vi "MIMIC Commands Rev 3.vi"(6 "MIMIC HOST COMMAND":T2(ring)=enum."Read Serial Number", 8 "Input String Data Array":string[](array[string])=["1"], 9 "HWHSflag":bool, 10 "wait (ms)":u32=500, 11 "VISA resource name":refnum<visa-resource-name>="COM5") -> (0 "error out":errorcluster={"status"=FALSE, "code"=1073676294, "source"="VISA Read in MIMIC RecvCommand.vi->MIMIC Commands Rev 2.vi"}, 1 "Receive_buffer":u8[](array[numeric]) format="%x", 2 "Receive_Unpacked_Data":T1)   [LabVIEW 2014]
panel:
  out "Array 2":u8[](array[numeric])
  out "Array":u8[](array[numeric])
  out "TimeToDecode":u16
  out "VISA resource name OUT":refnum<visa-resource-name>="COM5"
  out "hex integer string":string[](array[string])=["4", "D0", "0", "0", "FF", "2C"]
types:
  T1 = cluster{"Code_Revision":string, "Decode_Data":string, "Decode_Status":string, "Response_String_1":string, "Response_String_2":string, "Response_String_3":string, "Response_String_4":string, "Response_String_5":string, "Response_String_6":string, "Time_To_Decode":u16}
  T2 = enum16{"Enter FAT", "Beeper Control", "LED Off", "LED On", "Image Mode", "Start Session", "Stop Session", "Change Buadrate", "Auto Exposure", "Set Manual Exposure", "Read BT Address", "Store BT Address", "Pairing Command", "Query Paired Address", "Pairing Status", "Un-Pairing", "Set Illumination", "Trigger", "Set Defaults", "Imager Time To Decode Test", "Battery Off", "Battery Charge Control", "Read Battery Voltage", "Read Battery Temperature", "Software Version", "StoreFeatureSet", "ReadFeatureSet", "Store Model Number", "Read Model Number", "Store Manufacturing Date", "Read Manufacturing Date", "Store Service Date", "Read Service Date", "Store Serial Number", "Read Serial Number", "Exit FAT", "Read GUID", "Cable Auto ID", "Store RSM 627", "Read RSM 627", "Hall Effect switch", "ReadObjectSensor_AD", "Store_IR_Calibration", "Read_IR_Calibration", "Aim On", "Aim Off"}
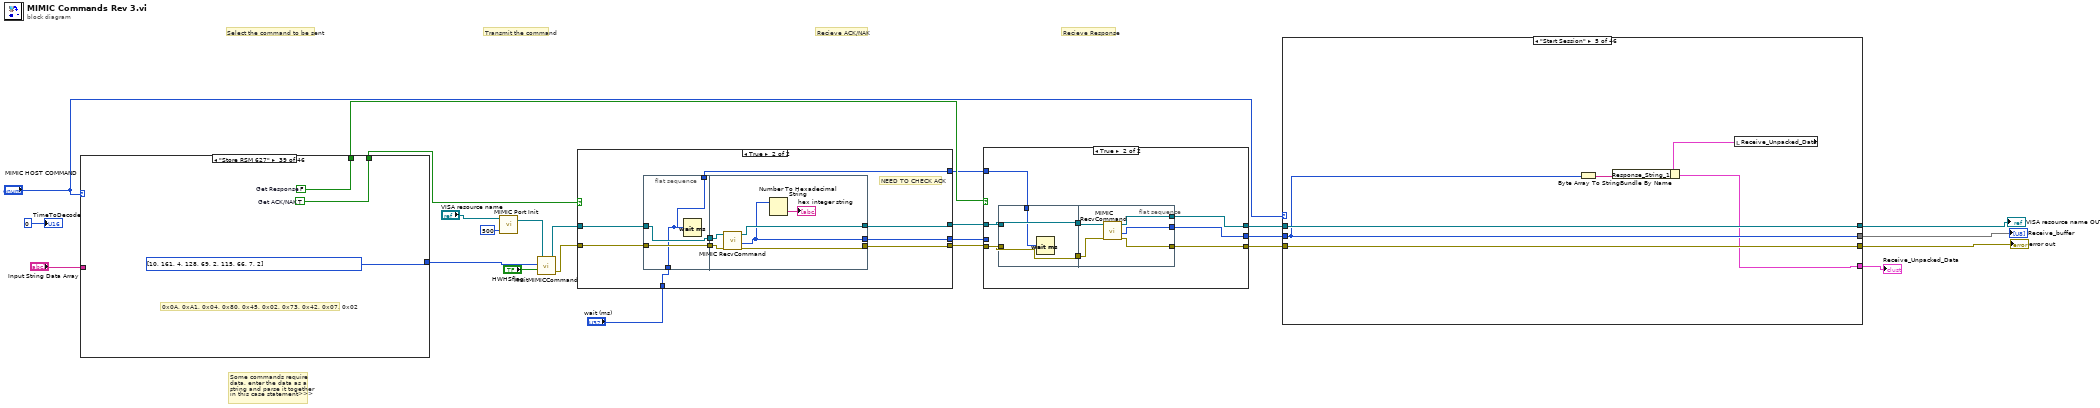
[diagram p0: block diagram]
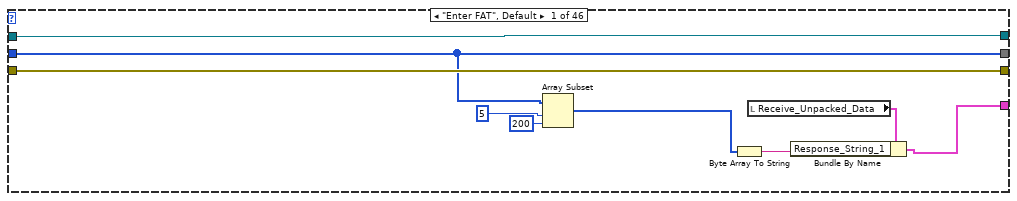
[diagram p2: hidden frame]
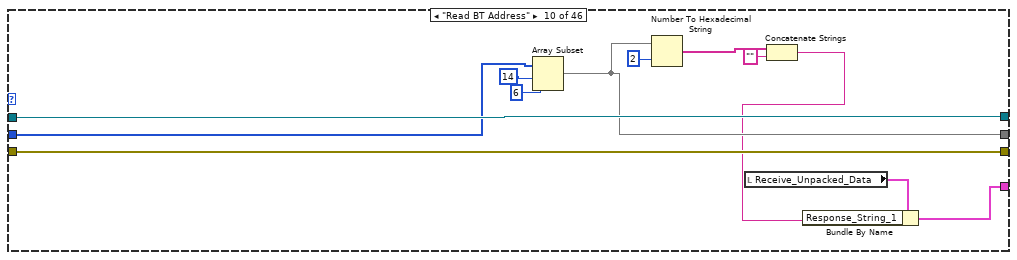
[diagram p10: hidden frame]
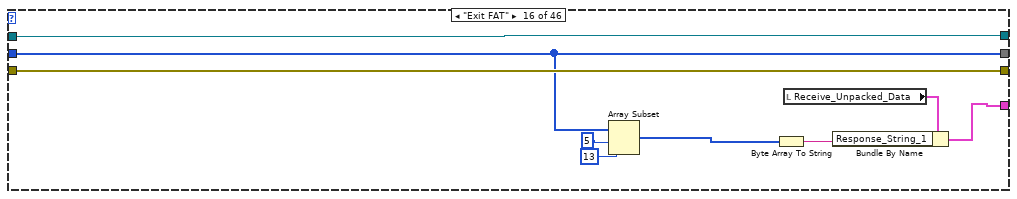
[diagram p16: hidden frame]
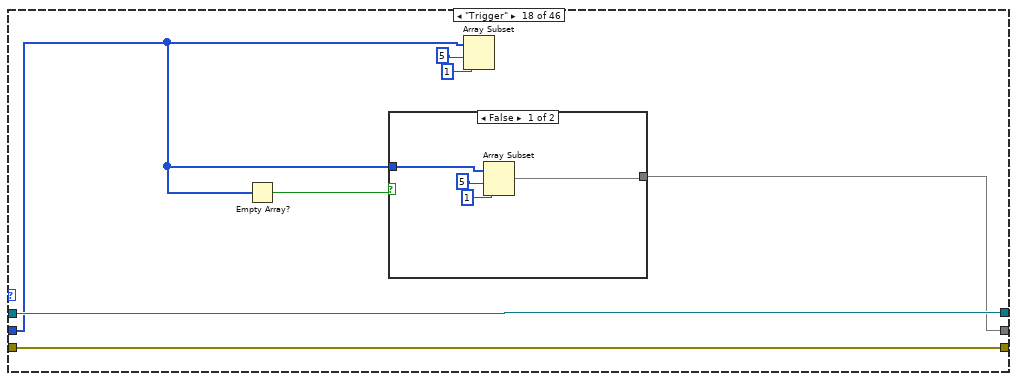
[diagram p18: hidden frame]
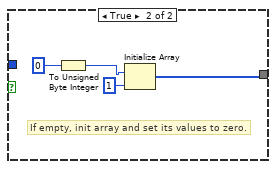
[diagram p19: hidden frame]
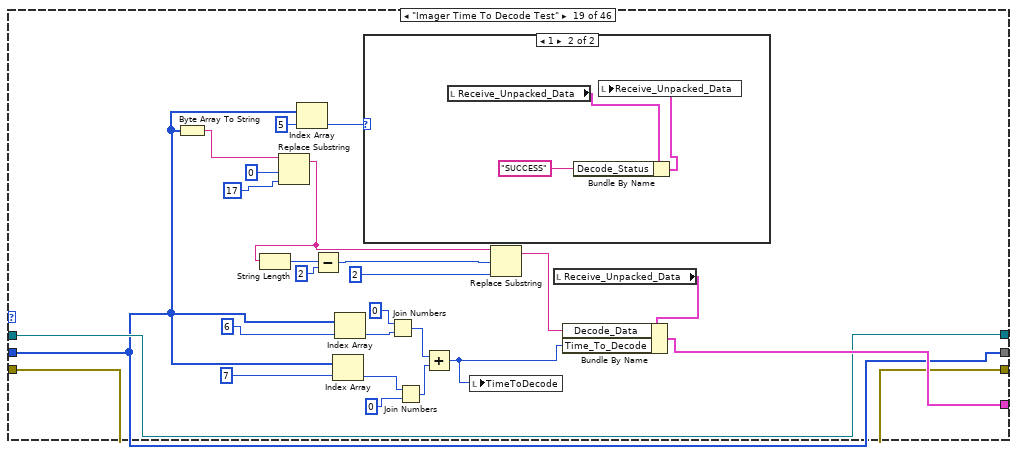
[diagram p20: hidden frame]
diagram:
  # "Transmit the command"
  # "Recieve Response"
  # "Recieve ACK/NAK"
  # "Select the command to be sent"
  # "Some commands require\ndata, enter the data as a\nstring and parse it together\nin this case statement>>>"
  n1 = case shown="\"Store RSM 627\"" "MIMIC HOST COMMAND" {
    tunnel: "Input String Data Array" -> [w33 w34 _ w45 _ _ _ w63 w79 w89 w102 _ _ _ _ _ w126 _ _ _ w146 _ _ _ w163 _ w173 _ _ _ w199 _ w211 _ _ _ _ _ _ _ _ _ w246 _ _ _]
    tunnel: [w27 w38 u8[] [5, 161, 4, 128, 16, 0, 0, 0, 0, 0, 0, 0, 0, 0] w46 u8[] [4, 228, 4, 0, 0, 0, 0, 0, 0, 0, 0, 0, 0, 0] u8[] [4, 228, 4, 0, 0, 0, 0, 0, 0, 0, 0, 0, 0, 0] u8[] [7, 215, 4, 0, 4, 11, 0, 255, 15, 0, 0, 0, 0, 0] w64 w73 w87 w101 u8[] [16, 161, 4, 128, 16, 0, 0, 0, 0, 0, 0, 0, 0, 0] u8[] [5, 161, 4, 128, 16, 0, 0, 0, 0, 0, 0, 0, 0, 0] u8[] [4, 200, 4, 128, 0, 0, 0, 0, 0, 0, 0, 0, 0, 0] u8[] [5, 161, 4, 128, 25, 0, 0, 0, 0, 0, 0, 0, 0, 0] u8[] [7, 161, 4, 128, 66, 2, 29, 0, 0, 0, 0, 0, 0, 0] w125 u8[] [6, 161, 4, 128, 45, 2, 0, 0, 0, 0, 0, 0, 0, 0] u8[] [7, 161, 4, 128, 48, 19, 136, 0, 0, 0, 0, 0, 0, 0] u8[] [5, 161, 4, 128, 60, 0, 0, 0, 0, 0, 0, 0, 0, 0] w145 u8[] [7, 161, 4, 128, 66, 117, 48, 0, 0, 0, 0, 0, 0, 0] u8[] [7, 161, 4, 128, 66, 117, 49, 0, 0, 0, 0, 0, 0, 0] u8[] [7, 161, 4, 128, 66, 78, 41, 0, 0, 0, 0, 0, 0, 0] w165 u8[] [7, 161, 4, 128, 66, 2, 194, 0, 0, 0, 0, 0, 0, 0] w178 u8[] [7, 161, 4, 128, 66, 2, 21, 0, 0, 0, 0, 0, 0, 0] w192 u8[] [7, 161, 4, 128, 66, 2, 23, 0, 0, 0, 0, 0, 0, 0] w204 u8[] [7, 161, 4, 128, 66, 2, 24, 0, 0, 0, 0, 0, 0, 0] w216 u8[] [7, 161, 4, 128, 66, 2, 22, 0, 0, 0, 0, 0] u8[] [5, 161, 4, 128, 54, 254, 160, 0, 0, 0, 0, 0, 0, 0] u8[] [5, 161, 4, 128, 84, 0, 0, 0, 0, 0, 0, 0, 0, 0] u8[] [5, 161, 4, 128, 47] u8[] [5, 161, 4, 128, 110] u8[] [10, 161, 4, 128, 69, 2, 115, 66, 7, 2] u8[] [6, 161, 4, 128, 45, 1, 0, 0, 0, 0, 0, 0, 0, 0] u8[] [7, 161, 4, 128, 66, 2, 115] u8[] [6, 161, 4, 128, 96, 8] w247 u8[] [7, 161, 4, 128, 66, 3, 36] u8[] [4, 197, 4, 128] u8[] [4, 196, 4, 128]] -> w19
    tunnel: [w26 w36 w43 w47 w55 w58 w60 w65 w80 w90 w108 w111 w113 w116 w120 w124 w128 w135 w139 w142 w143 w154 w157 w159 w168 w171 w177 w182 w191 w196 w203 w207 w214 w219 w223 w227 w228 w231 w234 w237 w241 w245 w249 w263 w266 w269] -> w21
    tunnel: [w25 w37 w42 w48 w56 w59 w61 w66 w81 w91 w109 w112 w114 w117 w119 w123 w127 w136 w138 w141 w144 w153 w156 w158 w167 w170 w176 w183 w190 w195 w202 w208 w215 w220 w222 w226 w229 w232 w235 w238 w240 w244 w248 w262 w265 w268] -> w23
    frame "LED On" {
      w26 = FALSE  # Get Response
      w25 = TRUE  # Get ACK/NAK
      # "LED data Byte"
      n2 = Index Array(array=w33, index=0) -> (element=w32:string)
      n3 = Decimal String To Number(string=w32) -> (number=w31:i32)  [unwired: 2 in, 1 out]
      n4 = Replace Array Subset(array=u8[] [5, 231, 4, 128, 1, 0, 0, 0, 0, 0, 0, 0, 0, 0], new element=w31, index=4) -> (w27:u8[])
    }
    frame "Beeper Control" {
      w36 = FALSE  # Get Response
      w37 = FALSE  # Get ACK/NAK
      # "Beeper data Byte"
      n5 = Decimal String To Number(string=w34, offset=0) -> (number=w41:i32[])  [unwired: 1 in, 1 out]
      n6 = Replace Array Subset(array=u8[] [5, 230, 4, 128, 0, 0, 0, 0, 0, 0, 0, 0, 0, 0], new element=w41, index=4) -> (w38:u8[])
    }
    frame "Enter FAT" {
      w43 = TRUE  # Get Response
      w42 = TRUE  # Get ACK/NAK
      # "Enter FAT command:\n0x05:0xA1:0x40:0x80:0x10"
    }
    frame "Image Mode" {
      w47 = FALSE  # Get Response
      w48 = TRUE  # Get ACK/NAK
      # "Image Mode Byte:\n00: Decode\n01: SnapShot\n02: Video\n03: Last Decode\n04: las No Decode"
      n7 = Index Array(array=w45, index=0) -> (element=w53:string)
      n8 = Decimal String To Number(string=w53) -> (number=w52:i32)  [unwired: 2 in, 1 out]
      n9 = Replace Array Subset(array=u8[] [5, 247, 4, 128, 0, 0, 0, 0, 0, 0, 0, 0, 0, 0], new element=w52, index=4) -> (w46:u8[])
    }
    frame "Start Session" {
      w55 = TRUE  # Get Response
      w56 = TRUE  # Get ACK/NAK
      # "Start Session"
    }
    frame "Stop Session" {
      w58 = FALSE  # Get Response
      w59 = TRUE  # Get ACK/NAK
      # "Start Session"
    }
    frame "Change Buadrate" {
      w60 = FALSE  # Get Response
      w61 = FALSE  # Get ACK/NAK
      # "Enter FAT command:\n06: 9600\n08: 38400\n0A: 57600\n0B:115200\n0C:230400"
    }
    frame "Auto Exposure" {
      w65 = FALSE  # Get Response
      w66 = TRUE  # Get ACK/NAK
      # "Auto Exposure:\n00:Disabled\n01: Enabled"
      n10 = Index Array(array=w63, index=0) -> (element=w71:string)
      n11 = Decimal String To Number(string=w71) -> (number=w70:i32)  [unwired: 2 in, 1 out]
      n12 = Replace Array Subset(array=u8[] [8, 198, 4, 0, 255, 240, 41, 0, 0, 0, 0, 0, 0, 0], new element=w70, index=7) -> (w64:u8[])
    }
    frame "Set Manual Exposure" {
      w80 = FALSE  # Get Response
      w81 = TRUE  # Get ACK/NAK
      # "Image Mode Byte:\n00: Decode\n01: SnapShot\n02: Video\n03: Last Decode\n04: las No Decode"
      n13 = Index Array(array=w79, index=0) -> (element=w85:string)
      n14 = Decimal String To Number(string=w85, default (0L)=u16 0 ("default (0 I32)")) -> (number=w78:u16)  [unwired: 1 in, 1 out]
      n15 = Split Number(x=w78) -> (hi(x)=w76:u8, lo(x)=w75:u8)
      n16 = Replace Array Subset(array=u8[] [10, 198, 4, 0, 255, 244, 241, 55, 0, 0, 0, 0, 0, 0], new element=w76, index=8) -> (w72:u8[])
      n17 = Replace Array Subset(array=w72, new element=w75, index=9) -> (w73:u8[])
    }
    frame "Store BT Address" {
      w90 = FALSE  # Get Response
      w91 = TRUE  # Get ACK/NAK
      # "Store BT command:\n0x16, 0xA1, 0x04, 0x80, 0x45, 0x02, 0x1D, 0x41, 0x07, 0x42, 0x00, 0x06, 0x00, 0x00, \n\t\t\t\t\t\t\t\t\t\t0x00, 0x00, 0x00, 0x00, 0x00, 0x00,0x00, 0x00, 0xFF, 0xFF};"
      n18 = for {
        N: 6 -> [_]
        tunnel: w89 -> [w100]
        tunnel: [w95] -> w87
        i -> [w97]
        n19 = Index Array(array=w100, index=w97) -> (element=w94:string)
        n20 = Add(x=14 ("index"), y=w97) -> (x+y=w98:i32)
        n21 = Hexadecimal String To Number(string=w94, offset=0) -> (number=w92:u32)  [unwired: 1 in, 1 out]
        n22 = local read "Array"() -> (w96:u8[])
        n23 = Replace Array Subset(array=w96, new element=w92, index=w98) -> (w95:u8[])
        n24 = local write "Array"(w95) -> ()
      }
      "Array" <- u8[] [22, 161, 4, 128, 69, 2, 29, 65, 7, 66, 0, 6, 0, 0, 0, 0, 0, 0, 0, 0, 255, 255, 255, 0, 0, 0]
    }
    frame "Pairing Command" {
      w108 = TRUE  # Get Response
      w109 = FALSE  # Get ACK/NAK
      # "Pairing  command:\n10 9E 04 80 00 00 02 03 06 08  01 0B 03 00 0F 0F FE 8E"
      n25 = Index Array(array=w102, index=0) -> (element=w106:string)
      n26 = String To Byte Array(string=w106) -> (unsigned byte array=w104:u8[])
      n27 = Replace Array Subset(array=u8[] [16, 158, 4, 128, 0, 0, 0, 0, 0, 8, 1, 11, 3, 0, 15, 15], new element=w104, index=4) -> (w101:u8[])
    }
    frame "Un-Pairing" {
      w111 = TRUE  # Get Response
      w112 = FALSE  # Get ACK/NAK
      # "Enter FAT command:\n0x05:0xA1:0x40:0x80:0x10"
    }
    frame "Set Illumination" {
      w113 = TRUE  # Get Response
      w114 = FALSE  # Get ACK/NAK
      # "Enter FAT command:\n0x05:0xA1:0x40:0x80:0x10"
    }
    frame "Set Defaults" {
      w116 = FALSE  # Get Response
      w117 = TRUE  # Get ACK/NAK
    }
    frame "Exit FAT" {
      w120 = TRUE  # Get Response
      w119 = TRUE  # Get ACK/NAK
    }
    frame "Read BT Address" {
      w124 = TRUE  # Get Response
      w123 = FALSE  # Get ACK/NAK
    }
    frame "LED Off" {
      w128 = FALSE  # Get Response
      w127 = TRUE  # Get ACK/NAK
      # "LED data Byte"
      n28 = Index Array(array=w126, index=0) -> (element=w133:string)
      n29 = Decimal String To Number(string=w133) -> (number=w132:i32)  [unwired: 2 in, 1 out]
      n30 = Replace Array Subset(array=u8[] [5, 232, 4, 128, 1, 0, 0, 0, 0, 0, 0, 0, 0, 0], new element=w132, index=4) -> (w125:u8[])
    }
    frame "Trigger" {
      w135 = TRUE  # Get Response
      w136 = TRUE  # Get ACK/NAK
    }
    frame "Imager Time To Decode Test" {
      w139 = TRUE  # Get Response
      w138 = TRUE  # Get ACK/NAK
      # "Start Session"
    }
    frame "Battery Off" {
      w142 = FALSE  # Get Response
      w141 = TRUE  # Get ACK/NAK
      # "Enter FAT command:\n0x05:0xA1:0x40:0x80:0x10"
    }
    frame "Battery Charge Control" {
      w143 = FALSE  # Get Response
      w144 = TRUE  # Get ACK/NAK
      # "Battery Charge\n0x06, 0xA1, 0x04, 0x80, 0x3D\n0x00: Disable charging of battery\n0x01: Enable charging of battery\n0x02: Enable Slow charge (Hammer)"
      n31 = Index Array(array=w146, index=0) -> (element=w151:string)
      n32 = Decimal String To Number(string=w151) -> (number=w150:i32)  [unwired: 2 in, 1 out]
      n33 = Replace Array Subset(array=u8[] [6, 161, 4, 128, 61, 0, 0, 0, 0, 0, 0, 0, 0, 0], new element=w150, index=5) -> (w145:u8[])
    }
    frame "Read Battery Voltage" {
      w154 = TRUE  # Get Response
      w153 = FALSE  # Get ACK/NAK
      # "Read Battery Voltage command:\n0x07:0xA1:0x04:0x80:0x42:0x75:0x30"
    }
    frame "Read Battery Temperature" {
      w157 = TRUE  # Get Response
      w156 = FALSE  # Get ACK/NAK
      # "Read Battery Temperature command:\n0x07:0xA1:0x04:0x80:0x42:0x75:0x31"
    }
    frame "Software Version" {
      w159 = TRUE  # Get Response
      w158 = TRUE  # Get ACK/NAK
      # "Software Version command:\n\"0x07, 0xA1, 0x04, 0x80, 0x42, 0x4E, 0x29,\""
    }
    frame "StoreFeatureSet" {
      w168 = FALSE  # Get Response
      w167 = TRUE  # Get ACK/NAK
      # "Store Feature Set command:\n\"0x0A, 0xA1, 0x04, 0x80, 0x45, 0x02, 0xC2, 0x42, 0x07,\n0xFF,//Feature Set Value \n0x00, 0x00}; //checksum\""
      n34 = Hexadecimal String To Number(string=w163, offset=0) -> (number=w161:u32[])  [unwired: 1 in, 1 out]
      n35 = Replace Array Subset(array=u8[] [10, 161, 4, 128, 69, 2, 194, 66, 7, 0, 0, 0, 0, 0], new element=w161, index=9) -> (w165:u8[])
    }
    frame "ReadFeatureSet" {
      w171 = TRUE  # Get Response
      w170 = TRUE  # Get ACK/NAK
      # "0x07, 0xA1, 0x04, 0x80, 0x42, 0x02, 0xC2, 0x00, 0x00};"
      # "Read Feature Set command:\n0x07, 0xA1, 0x04, 0x80, 0x42, 0x02, 0xC2,"
    }
    frame "Store Model Number" {
      w177 = FALSE  # Get Response
      w176 = TRUE  # Get ACK/NAK
      # "StoreModel Number command:\n0x20, 0xA1, 0x04, 0x80, 0x45, 0x02, 0x15, 0x53, 0x07, 0x00, 0x12, 0x00, 0x00,\n\t\t\t\t\t\t\t\t\t\t0x00, 0x00, 0x00, 0x00, 0x00, 0x00, 0x00, 0x00, 0x00,\n\t\t\t\t\t\t\t\t\t\t0x00, 0x00, 0x00, 0x00, 0x00, 0x00, 0x00, 0x00, 0x00,\n\t\t\t\t\t\t\t\t\t\t0x00"
      n36 = Index Array(array=w173, index=0) -> (element=w174:string)
      n37 = String To Byte Array(string=w174) -> (unsigned byte array=w175:u8[])
      n38 = Replace Array Subset(array=u8[] [32, 161, 4, 128, 69, 2, 21, 83, 7, 0, 18, 0, 0, 0, 0, 0, 0, 0, 0, 0, 0, 0, 0, 0, 0, 0, 0, 0, 0, 0, 0, 0, 0], new element=w175, index=13) -> (w178:u8[])
    }
    frame "Read Model Number" {
      w182 = TRUE  # Get Response
      w183 = TRUE  # Get ACK/NAK
      # "ReadModel Number command:\n0x07, 0xA1, 0x04, 0x80, 0x42, 0x02, 0x15,"
    }
    frame "Store Manufacturing Date" {
      w191 = FALSE  # Get Response
      w190 = TRUE  # Get ACK/NAK
      # "Store Manufacturing Date command:\n0x15, 0xA1, 0x04, 0x80, 0x45, 0x02, 0x17, 0x53, 0x07, 0x00, 0x07, 0x00, 0x00,\n\t\t\t\t\t\t\t\t\t\t0x00, 0x00, 0x00, 0x00, 0x00, 0x00, 0x00,\n\t\t\t\t\t\t\t\t\t\t0x00"
      n39 = Get Date/Time In Seconds() -> (seconds since 1Jan1904=w189:timestamp)
      n40 = Format Date/Time String(time format string (%c)="%d%b%y", seconds (now)=w189, UTC format=FALSE) -> (date/time string=w185:string)
      n41 = To Upper Case(1:w185) -> (0:w184:string)
      n42 = String To Byte Array(string=w184) -> (unsigned byte array=w186:u8[])
      n43 = Replace Array Subset(array=u8[] [21, 161, 4, 128, 69, 2, 23, 83, 7, 0, 7, 0, 0, 0, 0, 0, 0, 0, 0, 0, 0, 0], new element=w186, index=13) -> (w192:u8[])
    }
    frame "Read Manufacturing Date" {
      w196 = TRUE  # Get Response
      w195 = TRUE  # Get ACK/NAK
      # "Read Feature Set command:\n0x07, 0xA1, 0x04, 0x80, 0x42, 0x02, 0x17,"
    }
    frame "Store Service Date" {
      w203 = FALSE  # Get Response
      w202 = TRUE  # Get ACK/NAK
      # "StoreService Date command:\n0x15, 0xA1, 0x04, 0x80, 0x45, 0x02, 0x18, 0x53, 0x07, 0x00, 0x07, 0x00, 0x00,\n\t\t\t\t\t\t\t\t\t\t0x00, 0x00, 0x00, 0x00, 0x00, 0x00, 0x00,\n\t\t\t\t\t\t\t\t\t\t0x00"
      n44 = Index Array(array=w199, index=0) -> (element=w201:string)
      n45 = String To Byte Array(string=w201) -> (unsigned byte array=w198:u8[])
      n46 = Replace Array Subset(array=u8[] [21, 161, 4, 128, 69, 2, 24, 83, 7, 0, 7, 0, 0, 0, 0, 0, 0, 0, 0, 0, 0, 0], new element=w198, index=13) -> (w204:u8[])
    }
    frame "Read Service Date" {
      w207 = TRUE  # Get Response
      w208 = TRUE  # Get ACK/NAK
      # "Read Service Date command:\n0x07, 0xA1, 0x04, 0x80, 0x42, 0x02, 0x18,"
    }
    frame "Store Serial Number" {
      w214 = FALSE  # Get Response
      w215 = TRUE  # Get ACK/NAK
      # "Store Serial Number command:\n0x1E, 0xA1, 0x04, 0x80, 0x45, 0x02, 0x16, 0x53, 0x07, 0x00, 0x10, 0x00, 0x00,\n\t\t\t\t\t\t\t\t\t\t0x00, 0x00, 0x00, 0x00, 0x00, 0x00, 0x00, 0x00,\n\t\t\t\t\t\t\t\t\t\t0x00, 0x00, 0x00, 0x00, 0x00, 0x00, 0x00, 0x00,\n\t\t\t\t\t\t\t\t\t\t0x00"
      n47 = Index Array(array=w211, index=0) -> (element=w213:string)
      n48 = String To Byte Array(string=w213) -> (unsigned byte array=w210:u8[])
      n49 = Replace Array Subset(array=u8[] [30, 161, 4, 128, 69, 2, 22, 83, 7, 0, 16, 0, 0, 0, 0, 0, 0, 0, 0, 0, 0, 0, 0, 0, 0, 0, 0, 0, 0, 0, 0, 0, 0], new element=w210, index=13) -> (w216:u8[])
    }
    frame "Read Serial Number" {
      w219 = TRUE  # Get Response
      w220 = TRUE  # Get ACK/NAK
      # "Read Serial Number command:\n0x07, 0xA1, 0x04, 0x80, 0x42, 0x02, 0x16,"
    }
    frame "Pairing Status" {
      w223 = TRUE  # Get Response
      w222 = FALSE  # Get ACK/NAK
      # "Read Serial Number command:\n0x05, 0xA1, 0x04, 0x80, 0x36, 0xFE, 0xA0,"
    }
    frame "Query Paired Address" {
      w227 = TRUE  # Get Response
      w226 = FALSE  # Get ACK/NAK
      # "Read Serial Number command:\n0x05, 0xA1, 0x04, 0x80, 0x54,"
    }
    frame "Read GUID" {
      w228 = TRUE  # Get Response
      w229 = TRUE  # Get ACK/NAK
      # "\"0x05, 0xA1, 0x04, 0x80, 0x2F,\""
    }
    frame "Cable Auto ID" {
      w231 = TRUE  # Get Response
      w232 = TRUE  # Get ACK/NAK
      # "0x05, 0xA1, 0x04, 0x00, 0x6E"
    }
    frame "Store RSM 627" {
      w234 = FALSE  # Get Response
      w235 = TRUE  # Get ACK/NAK
      # "0x0A, 0xA1, 0x04, 0x80, 0x45, 0x02, 0x73, 0x42, 0x07, 0x02"
    }
    frame "Hall Effect switch" {
      w237 = TRUE  # Get Response
      w238 = TRUE  # Get ACK/NAK
    }
    frame "Read RSM 627" {
      w241 = TRUE  # Get Response
      w240 = TRUE  # Get ACK/NAK
      # "\"0x07, 0xA1, 0x04, 0x80, 0x42,0x02,0x73\""
    }
    frame "ReadObjectSensor_AD" {
      w245 = TRUE  # Get Response
      w244 = TRUE  # Get ACK/NAK
      # "Get Object Sensor command:\n\"0x06,0xA1,0x04,0x80,0x60,0x08,\""
    }
    frame "Store_IR_Calibration" {
      w249 = FALSE  # Get Response
      w248 = TRUE  # Get ACK/NAK
      # "StoreIR Calibration command:\n\"0x0B,0xA1,0x04,0x80,0x45,0x03,0x24,0x57,0x07,\"+Locals.Object_sensor_CAL_str"
      n50 = for {
        N: 2 -> [_]
        tunnel: w246 -> [w260]
        tunnel: [w255] -> w247
        i -> [w257]
        n51 = Index Array(array=w260, index=w257) -> (element=w254:string)
        n52 = Add(x=9 ("index"), y=w257) -> (x+y=w258:i32)
        n53 = Hexadecimal String To Number(string=w254, offset=0) -> (number=w252:u32)  [unwired: 1 in, 1 out]
        n54 = local read "Array 2"() -> (w256:u8[])
        n55 = Replace Array Subset(array=w256, new element=w252, index=w258) -> (w255:u8[])
        n56 = local write "Array 2"(w255) -> ()
      }
      "Array 2" <- u8[] [11, 161, 4, 128, 69, 3, 36, 87, 7, 0, 0, 255, 255]
    }
    frame "Read_IR_Calibration" {
      w263 = TRUE  # Get Response
      w262 = TRUE  # Get ACK/NAK
      # "Get IR Calibration command:\n\"0x07,0xA1,0x04,0x80,0x42,0x03,0x24,\""
    }
    frame "Aim On" {
      w266 = FALSE  # Get Response
      w265 = TRUE  # Get ACK/NAK
      # "Aim On command:\n\"0x04, 0xC5, 0x04, 0x80,\""
    }
    frame "Aim Off" {
      w269 = FALSE  # Get Response
      w268 = TRUE  # Get ACK/NAK
      # "Aim Off 0xC4, 0x04, 0x80,\""
    }
  }
  n57 = call "MIMIC Port Init.vi"("MIMIC TIMEOUT"=u32 500, "MIMIC_PORT"="VISA resource name") -> ("MIMIC PORT RESOURCE"=w3:refnum<visa-resource-name>)  [unwired: 1 in, 1 out]
  n58 = call "XmitMIMICCommand.vi"("HWHSflag"="HWHSflag", "Command array"=w19, "VISA resource name"=w3) -> ("error out"=w17:errorcluster, "VISA resource name Out"=w16:refnum<visa-resource-name>)  [unwired: 1 in]
  n59 = case shown="True" w23 {
    tunnel: [w272 w276] -> w22
    tunnel: w17 -> [w272 w281]
    tunnel: w16 -> [w271 w279]
    tunnel: [w271 w277] -> w20
    tunnel: [_ w275] -> w11
    tunnel: [w270 w274] -> w10
    tunnel: "wait (ms)" -> [w270 w273]
    frame False {
    }
    frame True {
      # "NEED TO CHECK ACK"
      n60 = flat-sequence {
        tunnel: w281 -> [w284]
        tunnel: [w284] -> w280
        tunnel: w279 -> [w283]
        tunnel: [w283] -> w278
        tunnel: [w282] -> w274
        tunnel: w273 -> [w282]
        tunnel: w280 -> [w289]
        tunnel: w278 -> [w288]
        tunnel: [w287] -> w277
        tunnel: [w286] -> w276
        tunnel: [w285] -> w275
        frame #0 {
          n61 = Wait (ms)(milliseconds to wait=w282) -> ()  [unwired: 1 out]
        }
        frame #1 {
          n62 = call "MIMIC RecvCommand.vi"("error in"=w289, "VISA resource name"=w288) -> ("error out"=w286:errorcluster, "Receive_buffer"=w285:u8[], "VISA resource name OUT"=w287:refnum<visa-resource-name>)  [unwired: 2 in, 1 out]
          n63 = Number To Hexadecimal String(2:w285) -> (0:→"hex integer string":string[])  [unwired: 1 in]
        }
      }
    }
  }
  n64 = case shown="True" w21 {
    tunnel: [w293 w300] -> w12
    tunnel: w22 -> [w293 w295]
    tunnel: w20 -> [w292 w297]
    tunnel: [w291 w301] -> w13
    tunnel: [w292 w299] -> w14
    tunnel: w11 -> [w291 _]
    tunnel: w10 -> [_ w294]
    frame False {
    }
    frame True {
      n65 = flat-sequence {
        tunnel: [w304] -> w298
        tunnel: w297 -> [w304]
        tunnel: [w303] -> w296
        tunnel: w295 -> [w303]
        tunnel: w294 -> [w302]
        tunnel: [w309] -> w301
        tunnel: [w308] -> w300
        tunnel: [w307] -> w299
        tunnel: w298 -> [w305]
        tunnel: w296 -> [w306]
        frame #0 {
          n66 = Wait (ms)(milliseconds to wait=w302) -> ()  [unwired: 1 out]
        }
        frame #1 {
          n67 = call "MIMIC RecvCommand.vi"("error in"=w306, "VISA resource name"=w305) -> ("error out"=w308:errorcluster, "Receive_buffer"=w309:u8[], "VISA resource name OUT"=w307:refnum<visa-resource-name>)  [unwired: 2 in, 1 out]
        }
      }
    }
  }
  n68 = case shown="\"Start Session\"" "MIMIC HOST COMMAND" {
    tunnel: w14 -> [w317 w321 w324 w327 w333 w336 w339 w342 w345 w357 w360 w363 w366 w369 w372 w381 w384 w391 w410 w433 w436 w442 w444 w454 w460 w463 w467 w477 w488 w496 w499 w508 w510 w521 w532 w537 w555 w558 w561 w566 w579 w585 w588 w591 w597 w600]
    tunnel: [w317 w321 w324 w327 w333 w336 w339 w342 w345 w357 w360 w363 w366 w369 w372 w381 w384 w391 w410 w433 w436 w442 w444 w454 w460 w463 w467 w477 w488 w496 w499 w508 w510 w521 w532 w537 w555 w558 w561 w566 w579 w585 w588 w591 w597 w600] -> w8
    tunnel: w13 -> [w313 w320 w323 w326 w330 w335 w338 w341 w344 w355 w359 w362 w365 w368 w371 w373 w383 w386 w408 w432 w435 w438 w446 w455 w459 w464 w468 w474 w487 w493 w498 w505 w511 w517 w525 w534 w550 w557 w560 w563 w578 w581 w587 w590 w596 w599]
    tunnel: [w313 w320 w323 w326 w330 w335 w338 w341 w344 w350 w359 w362 w365 w368 w371 w373 w383 w385 w408 w432 w435 w437 w445 w452 w459 w461 w468 w472 w487 w490 w498 w503 w511 w513 w523 w536 w549 w557 w560 w562 w578 w580 w587 w589 w596 w599] -> w7
    tunnel: w12 -> [w318 w319 w322 w325 w332 w334 w337 w340 w343 w356 w358 w361 w364 w367 w370 w380 w382 w390 w411 w431 w434 w441 w443 w453 w458 w462 w469 w478 w486 w497 w500 w509 w512 w520 w533 w538 w554 w556 w559 w565 w577 w584 w586 w592 w595 w598]
    tunnel: [w318 w319 w322 w325 w332 w334 w337 w340 w343 w356 w358 w361 w364 w367 w370 w380 w382 w390 w411 w431 w434 w441 w443 w453 w458 w462 w469 w478 w486 w497 w500 w509 w512 w520 w533 w538 w554 w556 w559 w565 w577 w584 w586 w592 w595 w598] -> w6
    tunnel: [w315 _ _ _ w328 _ _ _ _ w351 _ _ _ _ _ w377 _ _ w413 _ _ _ _ w449 _ _ _ w470 w480 w491 _ w501 _ w515 w524 _ w547 _ _ _ _ _ _ _ _ _] -> w4
    frame "Enter FAT", Default {
      n69 = Array Subset(array=w313, index=5, length=200) -> (w312:u8[])
      n70 = Byte Array To String(unsigned byte array=w312) -> (string=w316:string)
      n71 = local read "Receive_Unpacked_Data"() -> (w314:T1)
      n72 = Bundle By Name(cluster=w314, "Response_String_1"=w316) -> (w315:T1)
    }
    frame "Beeper Control" {
    }
    frame "LED On" {
    }
    frame "Image Mode" {
    }
    frame "Start Session" {
      n73 = Byte Array To String(unsigned byte array=w330) -> (string=w331:string)
      n74 = local read "Receive_Unpacked_Data"() -> (w329:T1)
      n75 = Bundle By Name(cluster=w329, "Response_String_1"=w331) -> (w328:T1)
    }
    frame "Stop Session" {
    }
    frame "Change Buadrate" {
    }
    frame "Auto Exposure" {
    }
    frame "Set Manual Exposure" {
    }
    frame "Read BT Address" {
      n76 = Array Subset(array=w355, index=14, length=6) -> (w350:u8[])
      n77 = Number To Hexadecimal String(1:i16 2 ("width (-)"), 2:w350) -> (0:w348:string[])
      n78 = local read "Receive_Unpacked_Data"() -> (w352:T1)
      n79 = Concatenate Strings(w348, "" ("string")) -> (w347:string)
      n80 = Bundle By Name(cluster=w352, "Response_String_1"=w347) -> (w351:T1)
    }
    frame "Store BT Address" {
    }
    frame "Pairing Command" {
    }
    frame "Un-Pairing" {
    }
    frame "Set Illumination" {
    }
    frame "Set Defaults" {
    }
    frame "Exit FAT" {
      n81 = Array Subset(array=w373, index=5, length=13) -> (w374:u8[])
      n82 = Byte Array To String(unsigned byte array=w374) -> (string=w379:string)
      n83 = local read "Receive_Unpacked_Data"() -> (w378:T1)
      n84 = Bundle By Name(cluster=w378, "Response_String_1"=w379) -> (w377:T1)
    }
    frame "LED Off" {
    }
    frame "Trigger" {
      n85 = Empty Array?(array=w386) -> (empty?=w387:bool)
      n86 = case shown="False" w387 {
        tunnel: w386 -> [w393 _]
        tunnel: [w392 w399] -> w385
        frame False {
          n87 = Array Subset(array=w393, index=5, length=1) -> (w392:u8[])
        }
        frame True {
          # "If empty, init array and set its values to zero."
          n88 = To Unsigned Byte Integer(number=u8 0) -> (unsigned 8bit integer=w397:u8)
          n89 = Initialize Array(w397, 1 ("dimension size")) -> (w399:u8[])
        }
      }
      n90 = Array Subset(array=w386, index=5, length=1) -> ()  [unwired: 1 out]
    }
    frame "Imager Time To Decode Test" {
      n91 = Byte Array To String(unsigned byte array=w408) -> (string=w424:string)
      n92 = Replace Substring(2:17 ("length (len. of substring)"), 3:0 ("offset (0)"), 5:w424) -> (1:w419:string)  [unwired: 1 in, 1 out]
      n93 = String Length(string=w419) -> (length=w418:i32)
      n94 = Index Array(array=w408, index=5) -> (element=w421:u8)
      n95 = Subtract(x=w418, y=2) -> (x-y=w416:i32)
      n96 = Index Array(array=w408, index=7 ("length")) -> (element=w403:u8)
      n97 = Index Array(array=w408, index=6) -> (element=w406:u8)
      n98 = case shown="1" w421 {
        frame 0, Default {
          n99 = local read "Receive_Unpacked_Data"() -> (w425:T1)
          n100 = Bundle By Name(cluster=w425, "Decode_Status"="No Decode" ("Decode_Data")) -> (w426:T1)
          n101 = local write "Receive_Unpacked_Data"(w426) -> ()
        }
        frame 1 {
          n102 = local read "Receive_Unpacked_Data"() -> (w429:T1)
          n103 = Bundle By Name(cluster=w429, "Decode_Status"="SUCCESS" ("Decode_Data")) -> (w428:T1)
          n104 = local write "Receive_Unpacked_Data"(w428) -> ()
        }
      }
      n105 = Join Numbers(hi=u8 0, lo=w406) -> ((hi.lo)=w401:u16)
      n106 = Join Numbers(hi=w403, lo=u8 0 ("hi")) -> ((hi.lo)=w402:u16)
      n107 = Add(x=w401, y=w402) -> (x+y=w400:u16)
      n108 = local write "TimeToDecode"(w400) -> ()
      n109 = Replace Substring(2:2 ("length (len. of substring)"), 3:w416, 5:w419) -> (1:w414:string)  [unwired: 1 in, 1 out]
      n110 = local read "Receive_Unpacked_Data"() -> (w412:T1)
      n111 = Bundle By Name(cluster=w412, "Decode_Data"=w414, "Time_To_Decode"=w400) -> (w413:T1)
    }
    frame "Battery Off" {
    }
    frame "Battery Charge Control" {
    }
    frame "Read Battery Voltage" {
      # "Voltage (MSB_LSB *.0006*2)"
      # "RESPONSE\nLength Byte:\t0x0D\nOpcode Byte:\t0x21\nSource Byte:\t0x00\nStatus Byte:\t0x80\nSub-opcode Byte:\t0x42\nData Byte 1:\t0x75: Attribute MSB\nData Byte 2:\t0x30: Attribute LSB\nData Byte 3:\t0x57: Attribute is Word ('W') value\nData Byte 4:\t0x01\nData Byte 5:\t0xXX: Battery Voltage MSB\nData Byte 6:\t0xXX: Battery Voltage LSB\nData Byte 7:\t0xFF: Packet Termination\nData Byte 8:\t0xFF: Packet Termination\nChecksum High Byte:\t0xXX\nChecksum Low Byte:\t0xXX"
      n112 = Array Subset(array=w438, index=0, length=15) -> (w437:u8[])
    }
    frame "Read Battery Temperature" {
      # "RESPONSE\nLength Byte:\t0x0D\nOpcode Byte:\t0x21\nSource Byte:\t0x00\nStatus Byte:\t0x80\nSub-opcode Byte:\t0x42\nData Byte 1:\t0x75: Attribute MSB\nData Byte 2:\t0x31: Attribute LSB\nData Byte 3:\t0x57: Attribute is Word ('W') value\nData Byte 4:\t0x01\nData Byte 5:\t0xXX: Battery Temperature MSB\nData Byte 6:\t0xXX: Battery Temperature LSB\nData Byte 7:\t0xFF: Packet Termination\nData Byte 8:\t0xFF: Packet Termination\nChecksum High Byte:\t0xXX\nChecksum Low Byte:\t0xXX"
      n113 = Array Subset(array=w446, index=0, length=15) -> (w445:u8[])
    }
    frame "Software Version" {
      n114 = Array Subset(array=w455, index=13, length=18) -> (w452:u8[])
      n115 = Byte Array To String(unsigned byte array=w452) -> (string=w451:string)
      n116 = local read "Receive_Unpacked_Data"() -> (w450:T1)
      n117 = Bundle By Name(cluster=w450, "Code_Revision"=w451) -> (w449:T1)
    }
    frame "StoreFeatureSet" {
    }
    frame "ReadFeatureSet" {
      # "Feature Set Responce:\n0x0C, 0x21, 0x00, 0x00, 0x42, 0x02, 0xC2,0x42,0x01,\n\t\t\t\t\t\t\t\t\t\t\t  \t\t\t  0xff, //FEATURE-SET\n\t\t\t\t\t\t\t\t\t\t\t\t\t\t  0xff,0xff, // packet termination\n\t\t\t\t\t\t\t\t\t\t\t\t\t\t  0x00, 0x00}; //checksum"
      n118 = Array Subset(array=w464, index=9, length=1) -> (w461:u8[])
    }
    frame "Store Model Number" {
    }
    frame "Read Model Number" {
      n119 = Array Subset(array=w474, index=13, length=18) -> (w472:u8[])
      n120 = Byte Array To String(unsigned byte array=w472) -> (string=w473:string)
      n121 = local read "Receive_Unpacked_Data"() -> (w471:T1)
      n122 = Bundle By Name(cluster=w471, "Response_String_1"=w473) -> (w470:T1)
    }
    frame "Store Manufacturing Date" {
      n123 = Get Date/Time In Seconds() -> (seconds since 1Jan1904=w485:timestamp)
      n124 = Format Date/Time String(time format string (%c)="%d%b%y", seconds (now)=w485, UTC format=FALSE) -> (date/time string=w482:string)
      n125 = To Upper Case(1:w482) -> (0:w479:string)
      n126 = local read "Receive_Unpacked_Data"() -> (w481:T1)
      n127 = Bundle By Name(cluster=w481, "Response_String_1"=w479) -> (w480:T1)
    }
    frame "Read Manufacturing Date" {
      n128 = Array Subset(array=w493, index=13, length=7) -> (w490:u8[])
      n129 = Byte Array To String(unsigned byte array=w490) -> (string=w492:string)
      n130 = local read "Receive_Unpacked_Data"() -> (w489:T1)
      n131 = Bundle By Name(cluster=w489, "Response_String_1"=w492) -> (w491:T1)
    }
    frame "Store Service Date" {
    }
    frame "Read Service Date" {
      n132 = Array Subset(array=w505, index=13, length=7) -> (w503:u8[])
      n133 = Byte Array To String(unsigned byte array=w503) -> (string=w504:string)
      n134 = local read "Receive_Unpacked_Data"() -> (w502:T1)
      n135 = Bundle By Name(cluster=w502, "Response_String_1"=w504) -> (w501:T1)
    }
    frame "Store Serial Number" {
    }
    frame "Read Serial Number" {
      n136 = Array Subset(array=w517, index=13, length=16) -> (w513:u8[])
      n137 = Byte Array To String(unsigned byte array=w513) -> (string=w516:string)
      n138 = local read "Receive_Unpacked_Data"() -> (w514:T1)
      n139 = Bundle By Name(cluster=w514, "Response_String_1"=w516) -> (w515:T1)
    }
    frame "Query Paired Address" {
      # "Cradle BT Address"
      # "Pair Status\n0x00: Unpaired \n0x01: Paired"
      n140 = Array Subset(array=w525, index=6, length=6) -> (w528:u8[])
      n141 = Array Subset(array=w525, index=5, length=1) -> (w523:u8[])
      n142 = local read "Receive_Unpacked_Data"() -> (w522:T1)
      n143 = Byte Array To String(unsigned byte array=w528) -> (string=w529:string)
      n144 = Bundle By Name(cluster=w522, "Response_String_1"=w529) -> (w524:T1)
    }
    frame "Pairing Status" {
      # "Pairing Status\n0x00: Cradle is not paired\n0x01: Cradle is paired"
      n145 = Empty Array?(array=w534) -> (empty?=w535:bool)
      n146 = case shown="True" w535 {
        tunnel: w534 -> [w540 _]
        tunnel: [w539 w546] -> w536
        frame False {
          n147 = Array Subset(array=w540, index=5, length=1) -> (w539:u8[])
        }
        frame True {
          # "If empty, init array and set its values to zero."
          n148 = To Unsigned Byte Integer(number=u8 0) -> (unsigned 8bit integer=w544:u8)
          n149 = Initialize Array(w544, 1 ("dimension size")) -> (w546:u8[])
        }
      }
    }
    frame "Read GUID" {
      n150 = Array Subset(array=w550, index=5, length=32) -> (w549:u8[])
      n151 = Byte Array To String(unsigned byte array=w549) -> (string=w553:string)
      n152 = local read "Receive_Unpacked_Data"() -> (w548:T1)
      n153 = Bundle By Name(cluster=w548, "Response_String_1"=w553) -> (w547:T1)
    }
    frame "Cable Auto ID" {
    }
    frame "Store RSM 627" {
    }
    frame "Hall Effect switch" {
      n154 = Empty Array?(array=w563) -> (empty?=w564:bool)
      n155 = case shown="False" w564 {
        tunnel: w563 -> [w570 _]
        tunnel: [w569 w576] -> w562
        frame False {
          n156 = Array Subset(array=w570, index=5, length=1) -> (w569:u8[])
        }
        frame True {
          # "If empty, init array and set its values to zero."
          n157 = To Unsigned Byte Integer(number=u8 0) -> (unsigned 8bit integer=w574:u8)
          n158 = Initialize Array(w574, 1 ("dimension size")) -> (w576:u8[])
        }
      }
      n159 = Array Subset(array=w563, index=5, length=1) -> ()  [unwired: 1 out]
    }
    frame "Read RSM 627" {
    }
    frame "ReadObjectSensor_AD" {
      n160 = Array Subset(array=w581, index=5, length=2) -> (w580:u8[])
    }
    frame "Store_IR_Calibration" {
    }
    frame "Read_IR_Calibration" {
      n161 = Array Subset(array=w590, index=9, length=2) -> (w589:u8[])
    }
    frame "Aim On" {
    }
    frame "Aim Off" {
    }
  }
  "error out" <- w6
  "Receive_buffer" <- w7
  "VISA resource name OUT" <- w8
  "Receive_Unpacked_Data" <- w4
  "TimeToDecode" <- u16 0 ("TimeToDecode")
